vi "replace input.vi"(8 "error in (no error)":errorcluster, 9 "Previous Input":string, 10 "State_Equations in":string[](array[string]), 11 "New Input":string) -> (0 "error out":errorcluster, 3 "State_Equations out":string[](array[string]))   [LabVIEW 2025, in "Dynamic-System.lvclass"]
uses:
  Dynamic-System.lvclass
  Dynamic-System.lvclass/Dynamic-System.ctl
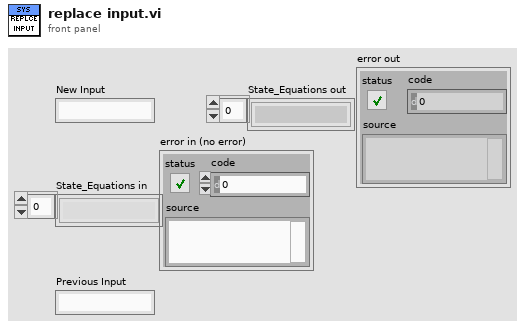
[diagram p1: front panel]
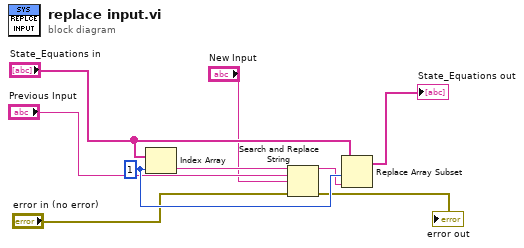
[diagram p0: block diagram]
diagram:
  w8 = 1 ("index")
  n1 = Index Array(array="State_Equations in", index=w8) -> (element=w5:string)
  n2 = Search and Replace String(input string=w5, search string="Previous Input", replace string="New Input", error in="error in (no error)") -> (result string=w7:string, error out=→"error out":errorcluster)  [unwired: 4 in, 2 out]
  n3 = Replace Array Subset(array="State_Equations in", new element=w7, index=w8) -> (→"State_Equations out":string[])
